vi "CameraConfig.vi"(7 "AOI":i32[](array[numeric]), 8 "error in":errorcluster, 9 "Caller Enqueuer":refnum<class "Message Enqueuer.lvclass">, 10 "ImageAcquisitionsParameters":T1={"Camera parameters"={"Id"=0, "Type"="", "Model"="", "InterfaceType"="", "SerialNumber"="", "Timeout"=0, "NumberOfBuffers"=0, "AcquisitionTimeout"=0, "ImageName"="", "ColorCameraParam"={"PixelFormat"="", "GammaEnable"=FALSE, "GammaSelector"="", "BalanceRationSelector"=[], "BalanceRationRaw"=[], "BalanceWhiteAuto"="", "LightSourceSelector"=""}, "sessionID"="", "Continuous?"=enum."One Shot", "Image Type"=0, "Buffer Number Mode (Next)"=enum."Next", "PartsList"=[{"Name"="", "ReceiverSequence"=[], "AOI"=[], "filePath"=""}], "AOI "=[], "Default file path"=path "", "Offline"=FALSE, "GeneralCameraConfig"=[], "DefaultReceiverSequence"=[], "Front Panel Open?"=FALSE}, "PartName"=[]} {"Camera parameters"."Image Type" items=["Grayscale (U8)", "Grayscale (I16)", "Grayscale (SGL)", "Complex (CSG)", "RGB (U32)", "HSL (U32)", "RGB (U64)", "Grayscale (U16)"]}, 11 "Session In":T2 caption="Session Out") -> (0 "error out":errorcluster, 3 "IMAQdx Session Out":T2)   [LabVIEW 2019, in "Image Acquisition.lvlib" / "Image Acquisition.lvclass"]
uses:
  Image Acquisition.lvclass
  <resource>/objmgr/imaqdx.rc
  <vilib>/userdefined/High Color/IMAQdx.ctl
  <vilib>/vision/driver/IMAQdx.llb/IMAQdx Buffer Number Mode.ctl
  <vilib>/vision/driver/IMAQdx.llb/IMAQdx Acquisition Mode.ctl
  <vilib>/ActorFramework/Message Enqueuer/Message Enqueuer.lvclass
  TypeDefs/Image Acquisition Parameters.ctl
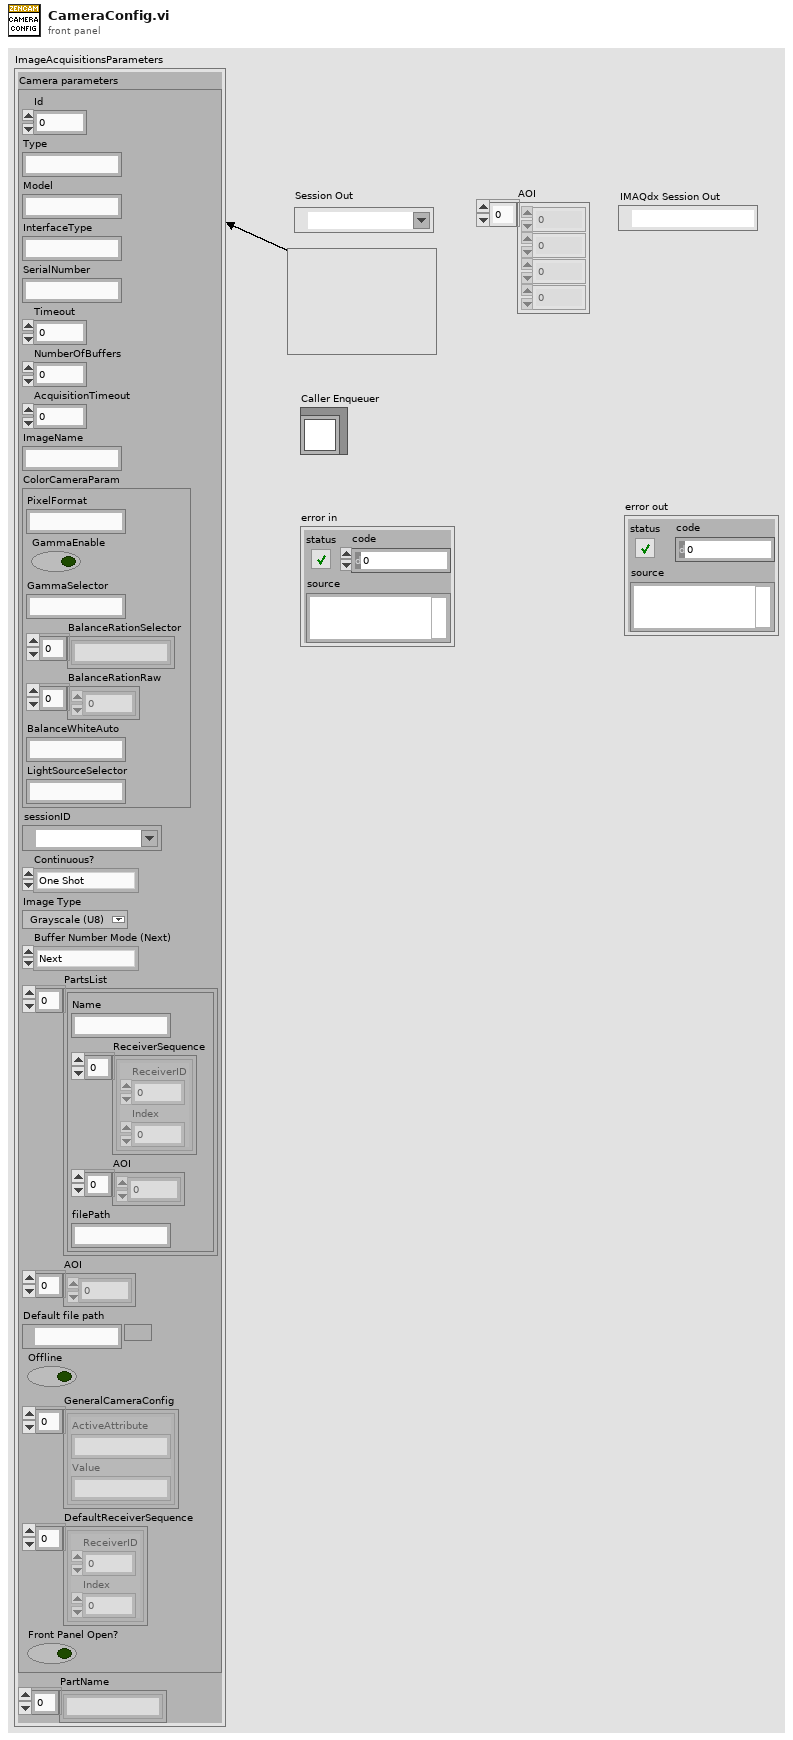
[diagram p1: front panel]
types:
  T1 = typedef "Image Acquisition.lvlib/Image Acquisition.lvclass/Image Acquisition Parameters.ctl" = cluster{"Camera parameters":cluster{"Id":i32, "Type":string, "Model":string, "InterfaceType":string, "SerialNumber":string, "Timeout":i32, "NumberOfBuffers":i32, "AcquisitionTimeout":i32, "ImageName":string, "ColorCameraParam":cluster{"PixelFormat":string, "GammaEnable":bool, "GammaSelector":string, "BalanceRationSelector":string[], "BalanceRationRaw":i32[], "BalanceWhiteAuto":string, "LightSourceSelector":string}, "sessionID":T2, "Continuous?":T3, "Image Type":T4, "Buffer Number Mode (Next)":T5, "PartsList":cluster{"Name":string, "ReceiverSequence":cluster{"ReceiverID":dbl, "Index":dbl}[], "AOI":i32[], "filePath":string}[], "AOI ":i32[], "Default file path":path, "Offline":bool, "GeneralCameraConfig":cluster{"ActiveAttribute":string, "Value":string}[], "DefaultReceiverSequence":cluster{"ReceiverID":dbl, "Index":dbl}[], "Front Panel Open?":bool}, "PartName":string[]}
  T2 = typedef "IMAQdx.ctl" = refnum<k21>
  T3 = typedef "NI_Vision_Acquisition_Software.lvlib/IMAQdx Acquisition Mode.ctl" = enum32{"One Shot", "Continuous"}
  T4 = typedef "Image Type" = u32
  T5 = typedef "NI_Vision_Acquisition_Software.lvlib/IMAQdx Buffer Number Mode.ctl" = enum32{"Next", "Last", "Buffer Number", "Every", "Last New"}
  T6 = cluster{"ActiveAttribute":string, "Value":string}[]
  T7 = cluster{"ActiveAttribute":string, "Value":string}
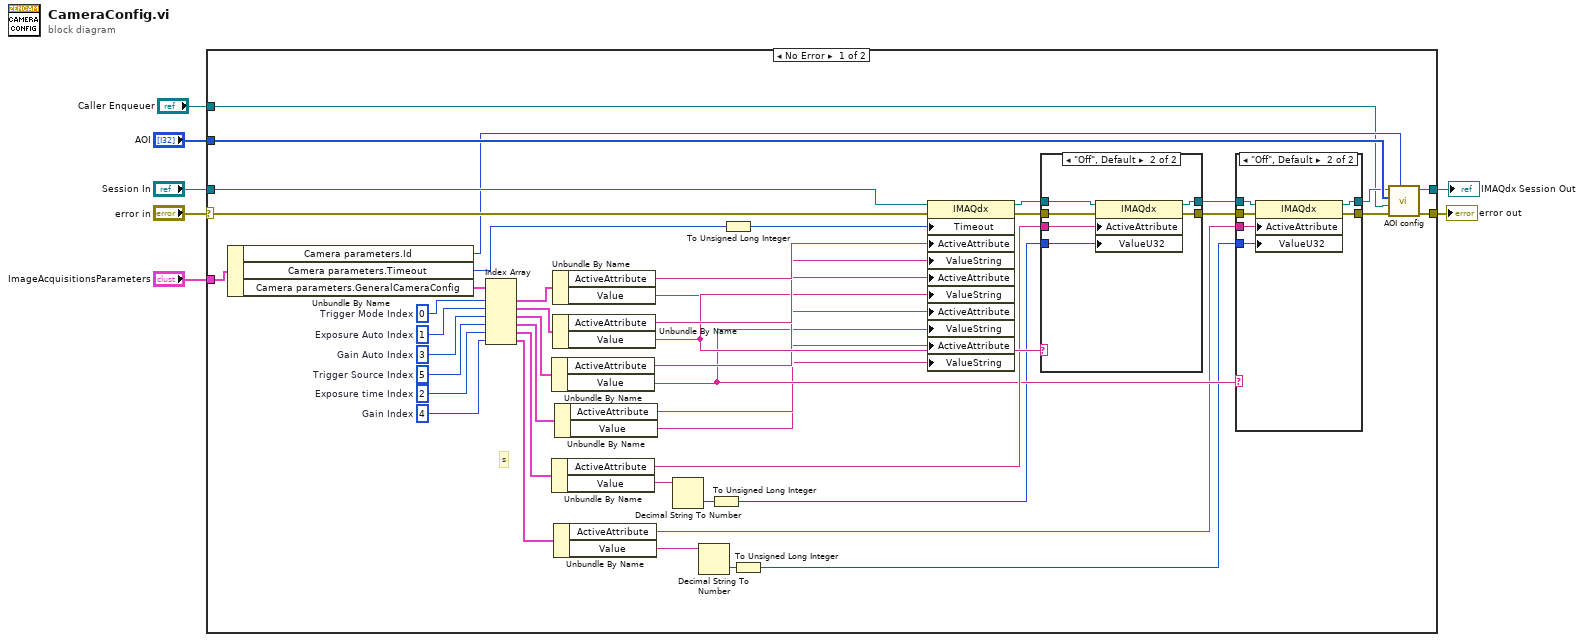
[diagram p0: block diagram]
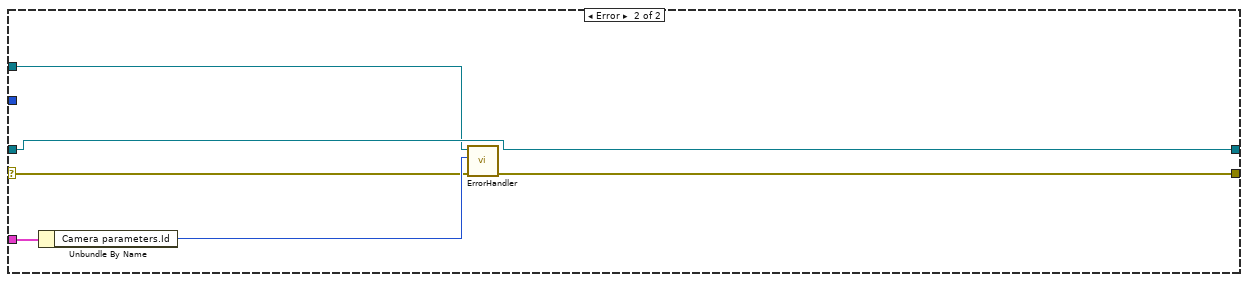
[diagram p4: hidden frame]
diagram:
  n1 = case shown="No Error" "error in" {
    selector: "error in" -> [w49 w69]
    tunnel: "Session In" -> [w52 w74]
    tunnel: "ImageAcquisitionsParameters" -> [w48 w73]
    tunnel: "AOI" -> [w47 _]
    tunnel: [w46 w74] -> w3
    tunnel: [w45 w70] -> w2
    tunnel: "Caller Enqueuer" -> [w17 w71]
    frame No Error {
      w10 = 5  # Trigger Source Index
      w12 = 4  # Gain Index
      w11 = 2  # Exposure time Index
      w20 = 3  # Gain Auto Index
      w21 = 1  # Exposure Auto Index
      w22 = 0  # Trigger Mode Index
      # "s"
      n2 = Unbundle By Name(w48) -> ("Camera parameters.Id"=w18:i32, "Camera parameters.Timeout"=w51:i32, "Camera parameters.GeneralCameraConfig"=w44:T6)
      n3 = Index Array(array=w44, index #1=w22, index #2=w21, index #3=w20, index #4=w10, index #5=w11, index #6=w12) -> (element #1=w43:T7, element #2=w41:T7, element #3=w19:T7, element #4=w13:T7, element #5=w14:T7, element #6=w15:T7)
      n4 = Unbundle By Name(w19) -> ("ActiveAttribute"=w30:string, "Value"=w28:string)
      n5 = Unbundle By Name(w14) -> ("ActiveAttribute"=w32:string, "Value"=w31:string)
      n6 = Unbundle By Name(w43) -> ("ActiveAttribute"=w42:string, "Value"=w29:string)
      n7 = Unbundle By Name(w41) -> ("ActiveAttribute"=w40:string, "Value"=w39:string)
      n8 = Unbundle By Name(w15) -> ("ActiveAttribute"=w27:string, "Value"=w26:string)
      n9 = Unbundle By Name(w13) -> ("ActiveAttribute"=w9:string, "Value"=w8:string)
      n10 = Decimal String To Number(string=w31) -> (number=w25:i32)  [unwired: 2 in, 1 out]
      n11 = Decimal String To Number(string=w26) -> (number=w16:i32)  [unwired: 2 in, 1 out]
      n12 = To Unsigned Long Integer(number=w25) -> (unsigned 32bit integer=w24:u32)
      n13 = To Unsigned Long Integer(number=w51) -> (unsigned 32bit integer=w50:u32)
      n14 = To Unsigned Long Integer(number=w16) -> (unsigned 32bit integer=w23:u32)
      n15 = property class="IMAQdx"(reference=w52, error in=w49, "Timeout"=w50, "ActiveAttribute"=w42, "ValueString"=w29, "ActiveAttribute"=w40, "ValueString"=w39, "ActiveAttribute"=w30, "ValueString"=w28, "ActiveAttribute"=w9, "ValueString"=w8) -> (reference out=w38:T2, error out=w37:errorcluster)
      n16 = case shown="\"Off\", Default" w39 {
        tunnel: w37 -> [w61 w68]
        tunnel: w38 -> [w62 w67]
        tunnel: [w62 w66] -> w35
        tunnel: [w61 w65] -> w36
        tunnel: w32 -> [_ w64]
        tunnel: w24 -> [_ w63]
        frame "Continuous" {
        }
        frame "Off", Default {
          n17 = property class="IMAQdx"(reference=w67, error in=w68, "ActiveAttribute"=w64, "ValueU32"=w63) -> (reference out=w66:T2, error out=w65:errorcluster)
        }
      }
      n18 = case shown="\"Off\", Default" w28 {
        tunnel: w36 -> [w53 w60]
        tunnel: w35 -> [w54 w59]
        tunnel: [w54 w58] -> w34
        tunnel: [w53 w57] -> w33
        tunnel: w27 -> [_ w56]
        tunnel: w23 -> [_ w55]
        frame "Continuous" {
        }
        frame "Off", Default {
          n19 = property class="IMAQdx"(reference=w59, error in=w60, "ActiveAttribute"=w56, "ValueU32"=w55) -> (reference out=w58:T2, error out=w57:errorcluster)
        }
      }
      n20 = call "AOI config.vi"("Camera parameters.Id"=w18, "error in (no error)"=w33, "Caller Enqueuer"=w17, "AOI"=w47, "IMAQdx in"=w34) -> ("error out"=w45:errorcluster, "IMAQdx out"=w46:T2)  [unwired: 5 in]
    }
    frame Error {
      n21 = Unbundle By Name(w73) -> ("Camera parameters.Id"=w72:i32)
      n22 = call "ErrorHandler.vi"("error in"=w69, "CameraID"=w72, "Caller Enqueuer"=w71) -> ("error out"=w70:errorcluster)  [unwired: 7 in, 1 out]
    }
  }
  "IMAQdx Session Out" <- w3
  "error out" <- w2
